vi "ma_Convert to dB.vi"(8 "dB reference (ch Y)":dbl=1.0 format="%0.2f", 9 "dB reference (ch X)":dbl=1.0 format="%0.2f", 10 "spectrum type":T1(ring), 11 "spectrum":dbl[](array[numeric]) format="%0.2f") -> (3 "spectrum in dB":dbl[](array[numeric]) format="%0.2f")   [LabVIEW 2020, in "NI_MAPro.lvlib"]
uses:
  NI_MAPro.lvlib
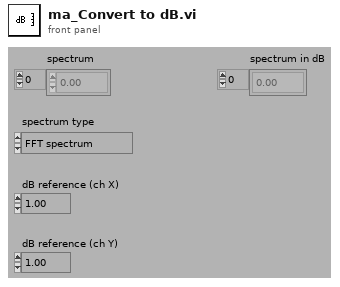
[diagram p1: front panel]
types:
  T1 = enum16{"FFT spectrum", "Power spectrum", "Cross spectrum", "Frequency response"}
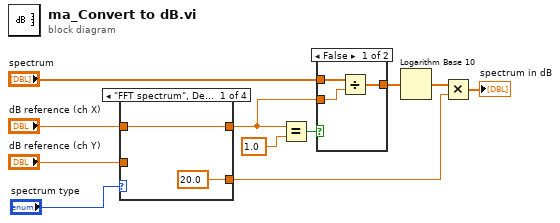
[diagram p0: block diagram]
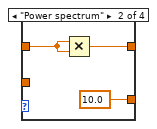
[diagram p2: hidden frame]
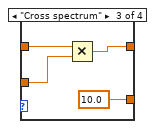
[diagram p3: hidden frame]
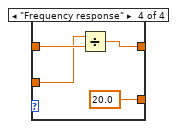
[diagram p4: hidden frame]
diagram:
  n1 = case shown="\"FFT spectrum\", Default" "spectrum type" {
    tunnel: "dB reference (ch X)" -> [w13 w15 w20 w24]
    tunnel: [w13 w16 w18 w23] -> w4
    tunnel: [20.0 ("y") 10.0 ("y") 10.0 ("y") 20.0 ("y")] -> w2
    tunnel: "dB reference (ch Y)" -> [_ _ w19 w22]
    frame "FFT spectrum", Default {
    }
    frame "Power spectrum" {
      n2 = Multiply(x=w15, y=w15) -> (x*y=w16:dbl)
    }
    frame "Cross spectrum" {
      n3 = Multiply(x=w20, y=w19) -> (x*y=w18:dbl)
    }
    frame "Frequency response" {
      n4 = Divide(x=w22, y=w24) -> (x/y=w23:dbl)
    }
  }
  n5 = Equal?(x=w4, y=1.0 ("dB reference")) -> (x = y?=w8:bool)
  n6 = case shown="False" w8 {
    tunnel: "spectrum" -> [w27 w28]
    tunnel: [w26 w28] -> w11
    tunnel: w4 -> [w25 _]
    frame False {
      n7 = Divide(x=w27, y=w25) -> (x/y=w26:dbl[])
    }
    frame True {
    }
  }
  n8 = Logarithm Base 10(1:w11) -> (0:w10:dbl[])
  n9 = Multiply(x=w10, y=w2) -> (x*y=→"spectrum in dB":dbl[])
